vi "Bad Action.vi"(8 "error in (no error)":errorcluster, 11 "Mouse in":refnum<class "Mouse.lvclass">) -> (0 "error out":errorcluster, 3 "Mouse out":refnum<class "Mouse.lvclass">)   [LabVIEW 2020, in "Maze.lvlib" / "Mouse.lvclass"]
doc: "This VI is called to let your mouse tried to take an action that wasn't possible. Your mouse either ran head-first into a wall, tried to drop a marker when one was already present, or tried picking up a marker when there wasn't one dropped. Once this VI is called the run is stopped. Overriding this VI can be useful for knowing when to reset class data that isn't helpful in completing a run."
uses:
  Mouse.lvclass
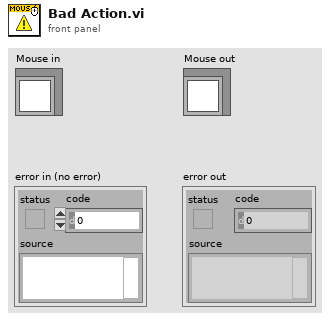
[diagram p1: front panel]
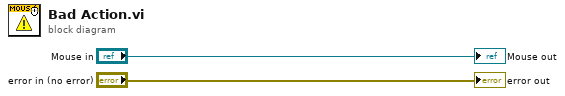
[diagram p0: block diagram]
diagram:
  "error out" <- "error in (no error)"
  "Mouse out" <- "Mouse in"
